vi "Stop Acquisition.vi"(8 "error in (no error)":errorcluster, 11 "Data Source in":refnum<class "Data Source.lvclass">) -> (0 "error out":errorcluster, 3 "Data Source out":refnum<class "Data Source.lvclass">)   [LabVIEW 2020, in "Data Source.lvlib" / "Data Source.lvclass"]
uses:
  Data Source.lvclass
  Data Source.lvclass/Data Source.ctl
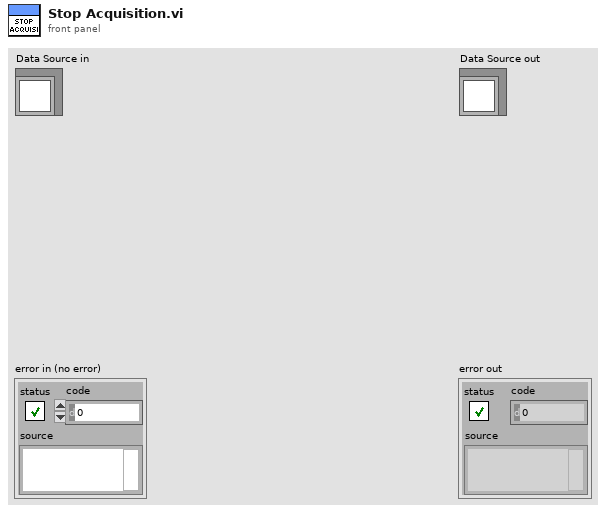
[diagram p1: front panel]
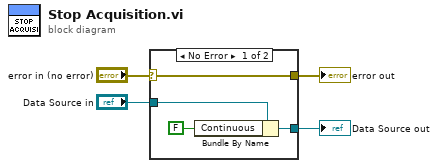
[diagram p0: block diagram]
diagram:
  n1 = case shown="No Error" "error in (no error)" {
    selector: "error in (no error)" -> [w8 w10]
    tunnel: [w8 w10] -> w3
    tunnel: [w6 w9] -> w1
    tunnel: "Data Source in" -> [w7 w9]
    frame No Error {
      n2 = Bundle By Name(cluster=w7, "Continuous"=FALSE) -> (w6:refnum<class "Data Source.lvclass">)
    }
    frame Error {
    }
  }
  "error out" <- w3
  "Data Source out" <- w1
